vi "Jiggle during modeshift.vi"(0 "Upper Limits":dbl[][](array[numeric])=[[0.0, 0.0583, 4.1], [3.2, 0.0583, 1.1]], 5 "Lower Limits":dbl[][](array[numeric])=[[0.0, 0.025, 3.8], [2.9, 0.025, 0.7]], 7 "Timeout (s)":dbl=60.0 format="%0.2f", 11 "Error In":errorcluster) -> (4 "Pass/Fail?":bool, 6 "Report Text":string, 8 "Results":dbl[][](array[numeric])=[[0.0, 0.042, 1.458], [0.542, 0.042, 0.916]], 15 "Error Out":errorcluster)   [LabVIEW 2016, in "Centauro.lvlib"]
uses:
  Projects/Centauro.lvlib
  <vilib>/DAQmx/read.llb/DAQmx Read (Digital 1D Wfm NChan NSamp).vi
  <vilib>/DAQmx/create/channels.llb/DAQmx Create Channel (DI-Digital Input).vi
  <vilib>/DAQmx/configure/timing.llb/DAQmx Timing (Sample Clock).vi
  <vilib>/DAQmx/configure/trigger.llb/DAQmx Start Trigger (Digital Edge).vi
  <vilib>/DAQmx/miscellaneous.llb/DAQmx Fill In Error Info.vi
panel:
  out "Digital Waveform Graph":digitalwaveform[](graph)
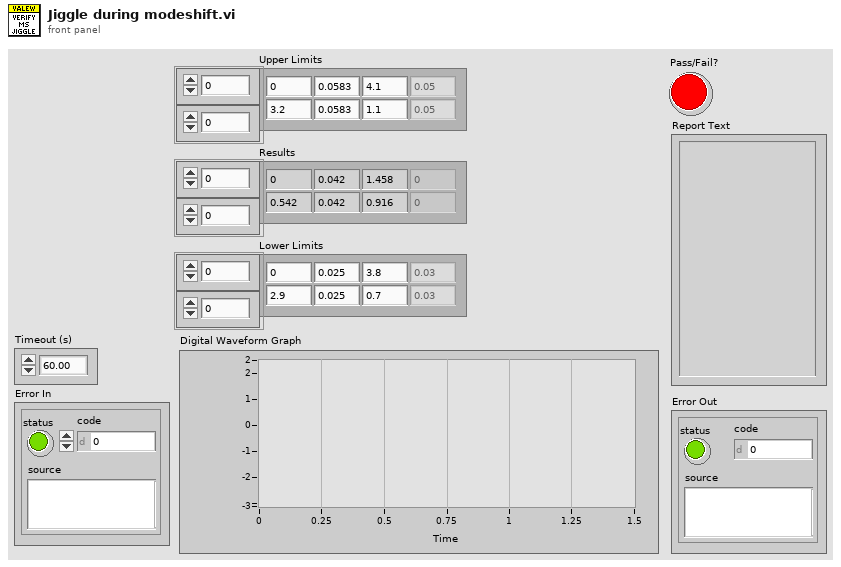
[diagram p1: front panel]
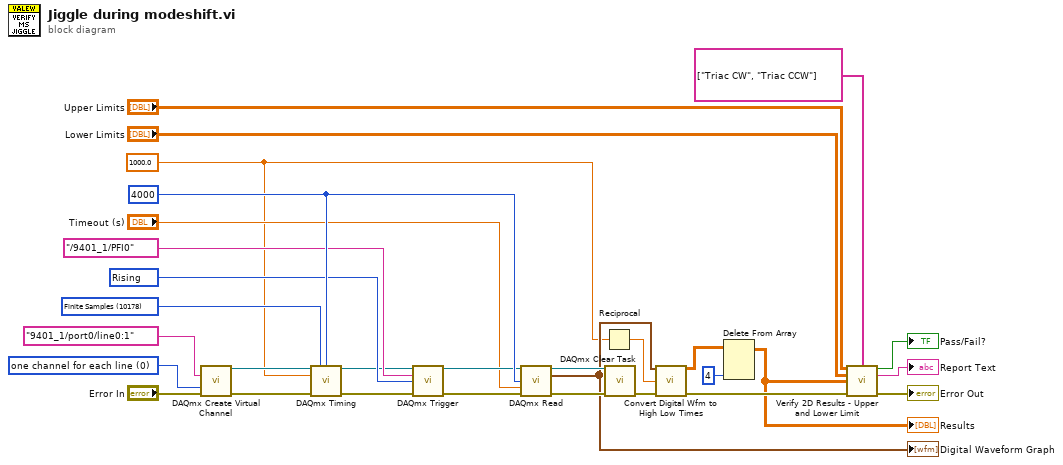
[diagram p0: block diagram]
diagram:
  w21 = 10280 items=["Rising"=10280, "Falling"=10171] ("edge")
  w26 = 0 items=["one channel for each line", "one channel for all lines"] ("line grouping")
  w14 = 1000.0 ("rate")
  w23 = 4000 ("samples per channel")
  w28 = 10178 items=["Finite Samples"=10178, "Continuous Samples"=10123, "Hardware Timed Single Point"=12522] ("sample mode")
  n1 = call-poly <vilib>:"DAQmx Create Virtual Channel.vi"("lines"=tag "9401_1/port0/line0:1", "line grouping"=w26, "error in"="Error In") -> ("task out"=w30:refnum<k21>, "error out"=w29:errorcluster)  [unwired: 11 in]
  n2 = call-poly <vilib>:"DAQmx Timing.vi"("task/channels in"=w30, "sample mode"=w28, "samples per channel"=w23, "rate"=w14, "error in"=w29) -> ("task out"=w20:refnum<k21>, "error out"=w18:errorcluster)  [unwired: 9 in]
  n3 = call-poly <vilib>:"DAQmx Trigger.vi"("task/channels in"=w20, "source"=tag "/9401_1/PFI0", "edge"=w21, "error in"=w18) -> ("task out"=w19:refnum<k21>, "error out"=w2:errorcluster)  [unwired: 10 in]
  n4 = call-poly <vilib>:"DAQmx Read.vi"("task/channels in"=w19, "number of samples per channel"=w23, "timeout"="Timeout (s)", "error in"=w2) -> ("task out"=w25:refnum<k21>, "data"=w16:digitalwaveform[], "error out"=w24:errorcluster)  [unwired: 9 in]
  "Digital Waveform Graph" <- w16
  n5 = Reciprocal(x=w14) -> (1/x=w15:dbl)
  n6 = call <vilib>:"DAQmx Clear Task.vi"("task in"=w25, "error in"=w24) -> ("error out"=w13:errorcluster)  [unwired: 13 in]
  n7 = call "Convert Digital Wfm to High Low Times.vi"("Digital Waveform In"=w16, "Dt"=w15, "Error In"=w13) -> ("HL Raw Output"=w7:dbl[][], "Error Out"=w12:errorcluster)  [unwired: 11 in]
  n8 = Delete From Array(array=w7, index (col)=4 ("disabled index (col)")) -> (array with subset deleted=w6:dbl[][])  [unwired: 2 in, 1 out]
  "Results" <- w6
  n9 = call "Verify 2D Results - Upper and Lower Limit.vi"("Upper Limits"="Upper Limits", "Array of Names"=string[] ["Triac CW", "Triac CCW"], "Lower Limits"="Lower Limits", "Results"=w6, "Error In"=w12) -> ("Pass/Fail?"=→"Pass/Fail?":bool, "Report Text"=→"Report Text":string, "Error Out"=→"Error Out":errorcluster)  [unwired: 7 in, 1 out]
